vi "read TBM configuration.vi"(8 "error in":errorcluster, 11 "Shared Library Module editor node in":refnum<class "Shared Library Module editor node.lvclass">) -> (0 "error out":errorcluster, 2 "TBM configuration out":refnum<class "TBM configuration.lvclass">, 3 "Shared Library Module editor node out":refnum<class "Shared Library Module editor node.lvclass">)   [LabVIEW 2013, in "Shared Library Module editor node.lvclass"]
doc: "Platypus Framework 1.0.1.60\nNI Systems Engineering - National Instruments"
uses:
  Shared Library Module editor node.lvclass
  <vilib>/NI/Tag Bus Module Framework/root configuration/TBM configuration.lvclass
  Shared Library Module editor node.lvclass/Shared Library Module editor node.ctl
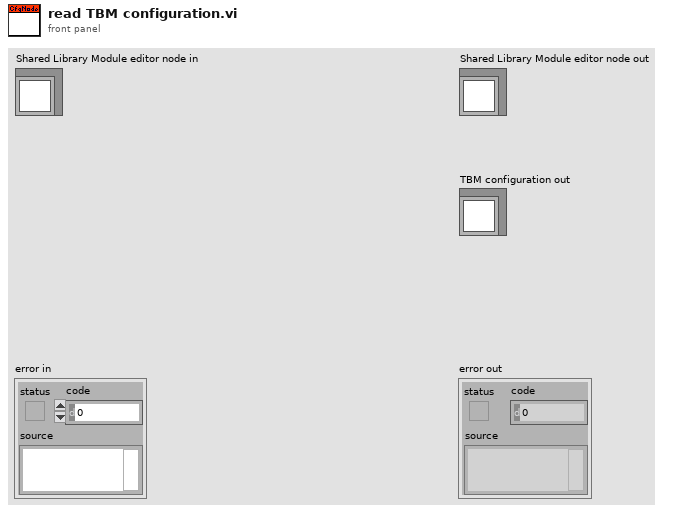
[diagram p1: front panel]
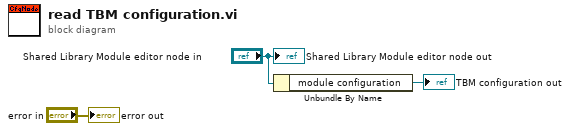
[diagram p0: block diagram]
diagram:
  n1 = Unbundle By Name("Shared Library Module editor node in") -> ("module configuration"=→"TBM configuration out":refnum<class "Shared Library Module configuration.lvclass">)
  "error out" <- "error in"
  "Shared Library Module editor node out" <- "Shared Library Module editor node in"
